vi "Configure Device.vi"(8 "error in":errorcluster, 11 "Device in":refnum<class "TE Cooler.lvclass">) -> (0 "error out":errorcluster, 3 "Device out":refnum<class "TE Cooler.lvclass">, 4 "SP":dbl, 5 "Settable?":bool)   [LabVIEW 2014, in "TE Cooler.lvlib" / "TE Cooler.lvclass"]
doc: "This is the configuration method for the Device object. The one parameter that all should have in common and is not dependent on the configuration of the device is the label which is read from the ini file. All devices that use this class should have this in their configuration."
uses:
  TE Cooler.lvclass
  reusable/Session APIs/Serial/Serial Session.lvclass
  Configurable Device/Configurable Device.lvclass/Configurable Device.ctl
  Configurable Device/Read Handle.vi
  Configurable Device/Accessors/Write type.vi
  Configurable Device/Accessors/Write controller_.vi
  Configurable Device/Read Log Session.vi
  reusable/Session APIs/File Access/Config Data/Config Data.lvclass
  <userlib>/_Session Fwk/Session - Root.lvclass
  reusable/Session APIs/Session Log/System Log.lvclass
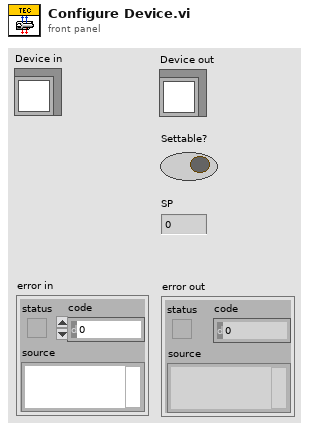
[diagram p1: front panel]
types:
  T1 = typedef "Serial Session.lvclass/Session Handle.ctl" = refnum<data-value>
  T2 = typedef "Config Data.lvclass/Config Session.ctl" = refnum<data-value>
  T3 = typedef "Session - Root.lvclass/Session Handle.ctl" = refnum<data-value>
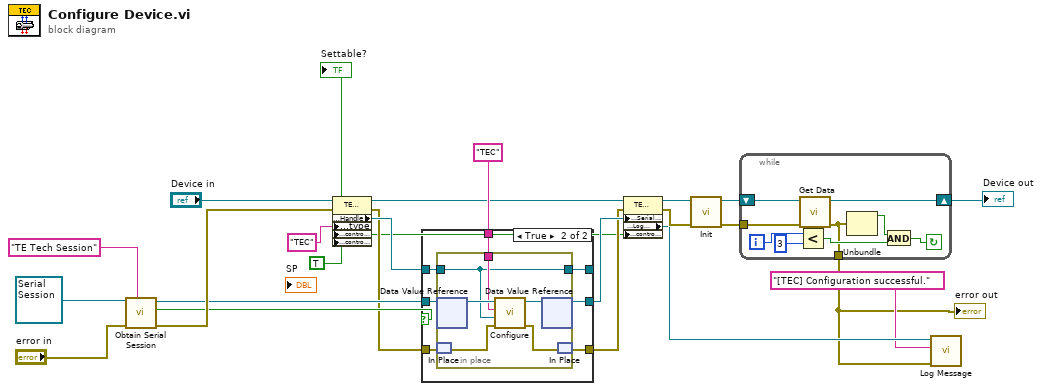
[diagram p0: block diagram]
diagram:
  w2 = TRUE ("controller_")
  n1 = call "Obtain Serial Session.vi"("Session Name ()"="TE Tech Session", "error in"="error in", "Serial Session in"=refnum<class "Serial Session.lvclass"> refnum) -> ("error out"=w20:errorcluster, "created new?"=w17:bool, "hSerial"=w16:T1)  [unwired: 6 in]
  n2 = property class="TE Tech"(reference="Device in", error in=w20, "Accessors:type"="TEC" ("type"), "Accessors:controller_"=w2, "Accessors:controller_"=w2) -> (reference out=w15:refnum<class "TE Cooler.lvclass">, error out=w7:errorcluster, "Accessors:Handle"=w18:T2)
  n3 = case shown="True" w17 {
    tunnel: w16 -> [w26 w33]
    tunnel: w7 -> [w25 w29]
    tunnel: [w26 w32] -> w14
    tunnel: [w25 w31] -> w6
    tunnel: w18 -> [w24 w30]
    tunnel: [w24 w28] -> _
    tunnel: "TEC" ("section") -> [_ w27]
    frame False {
    }
    frame True {
      n4 = in-place {
        in-place-border: w30 -> [w34]
        in-place-border: w27 -> [w35]
        in-place-border: [w34] -> w28
        n5 = in-place-dvr #1(w33) -> (w39:refnum<class "Serial Session.lvclass">)  [unwired: 1 out]
        n6 = in-place-match #2(w29) -> (w38:errorcluster)
        n7 = call "Configure.vi"("error in"=w38, "Config Handle"=w34, "section"=w35, "Serial Session in"=w39) -> ("error out"=w37:errorcluster, "Serial Session out"=w36:refnum<class "Serial Session.lvclass">)  [unwired: 6 in]
        n8 = in-place-dvr #1(w36) -> (w32:T1)  [unwired: 1 out]
        n9 = in-place-match #2(w37) -> (w31:errorcluster)
      }
    }
  }
  n10 = property class="TE Tech"(reference=w15, error in=w6, "Accessors:Serial Session"=w14, "Accessors:controller_"=w2) -> (reference out=w13:refnum<class "TE Cooler.lvclass">, error out=w12:errorcluster, "Accessors:Log Session"=w9:T3)
  n11 = call-dynamic "Init.vi"("error in"=w12, "TE Cooler in"=w13) -> ("error out"=w10:errorcluster, "TE Cooler out"=w11:refnum<class "TE Cooler.lvclass">)  [unwired: 8 in]
  n12 = while {
    shift-right: [w47] -> w4
    shift-left: w11 -> [w48]
    tunnel: [w41] -> w5
    tunnel: w10 -> [w40]
    i -> [w44]
    stop <- w45 continue-if-true
    n13 = Less?(x=w44, y=3) -> (x < y?=w42:bool)
    n14 = call-dynamic "Get Data.vi"("error in"=w40, "TE Cooler in"=w48) -> ("error out"=w41:errorcluster, "TE Cooler out"=w47:refnum<class "TE Cooler.lvclass">)  [unwired: 7 in, 1 out]
    n15 = Unbundle(w41) -> ("status"=w46:bool)  [unwired: 2 out]
    n16 = And(x=w46, y=w42) -> (x .and. y?=w45:bool)
  }
  "error out" <- w5
  "Device out" <- w4
  n17 = call "Log Message.vi"("error in"=w5, "MSG In"="[TEC] Configuration successful.", "session in"=w9) -> ()  [unwired: 7 in, 2 out]
  "Settable?" <- w2
